vi "WfmDataAccessor ReadData.vi"(8 "error in (no error)":errorcluster, 9 "Filename":string, 11 "WfmDataAccessor in":refnum<class "WfmDataAccessor.lvclass">) -> (0 "error out":errorcluster, 1 "WfmData":u64[](array[numeric]), 3 "WfmDataAccessor out":refnum<class "WfmDataAccessor.lvclass">)   [LabVIEW 2018, in "WfmDataAccessor.lvclass"]
uses:
  WfmDataAccessor.lvclass
  WfmDataAccessor.lvclass/WfmDataAccessor.ctl
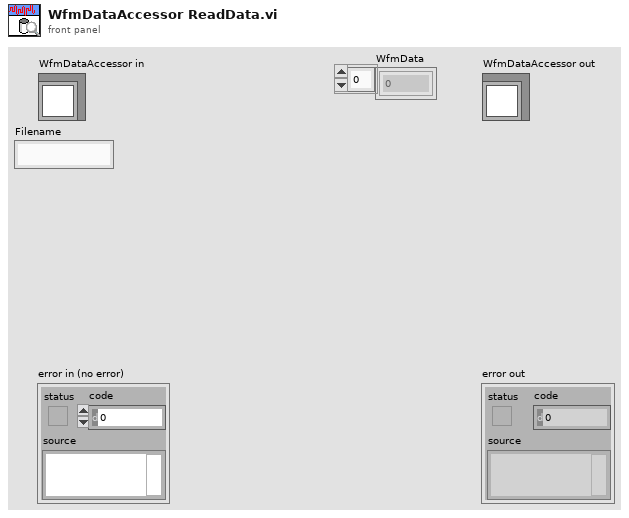
[diagram p1: front panel]
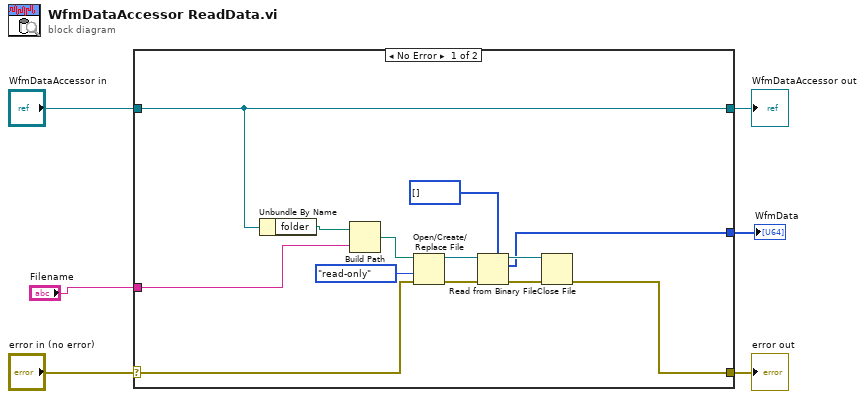
[diagram p0: block diagram]
diagram:
  n1 = case shown="No Error" "error in (no error)" {
    selector: "error in (no error)" -> [w15 w21]
    tunnel: [w8 w21] -> w5
    tunnel: [w19 w20] -> w3
    tunnel: "WfmDataAccessor in" -> [w19 w20]
    tunnel: "Filename" -> [w17 _]
    tunnel: [w7 _] -> w1
    frame No Error {
      n2 = Unbundle By Name(w19) -> ("folder"=w18:path)
      n3 = Build Path(base path=w18, name or relative path=w17) -> (appended path=w16:path)
      n4 = Open/Create/Replace File(file path (use dialog)=w16, error in=w15, access (0:read/write)=enum16{"read/write", "read-only", "write-only"}."read-only") -> (refnum out=w14:refnum<file>, error out=w13:errorcluster)  [unwired: 3 in, 1 out]
      n5 = Read from Binary File(5:u64[] [], 8:w13, 11:w14) -> (0:w9:errorcluster, 2:w7:u64[], 3:w10:refnum<file>)  [unwired: 3 in, 1 out]
      n6 = Close File(refnum=w10, error in=w9) -> (error out=w8:errorcluster)  [unwired: 1 out]
    }
    frame Error {
    }
  }
  "error out" <- w5
  "WfmDataAccessor out" <- w3
  "WfmData" <- w1
